vi "DataRootPathFGV.vi"(8 "Error In":errorcluster, 10 "action (write)":enum16{"write", "read"}(ring), 11 "PathIn":path) -> (0 "Error Out":errorcluster, 3 "PathOut":path)   [LabVIEW 2019]
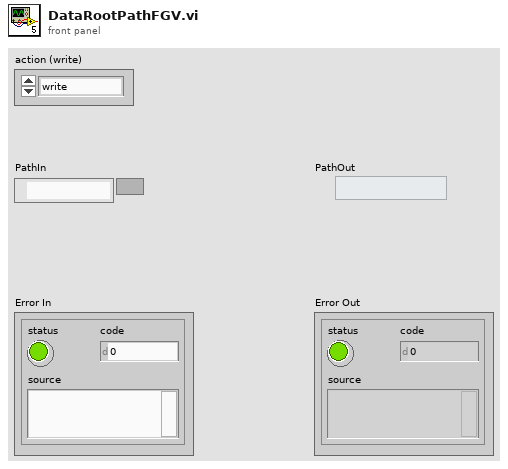
[diagram p1: front panel]
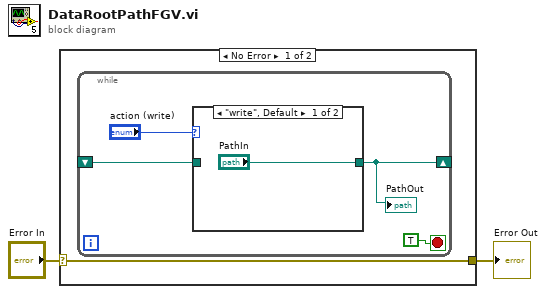
[diagram p0: block diagram]
diagram:
  n1 = case shown="No Error" "Error In" {
    selector: "Error In" -> [w3 w10]
    tunnel: [w3 w10] -> w1
    frame No Error {
      n2 = while {
        shift-right: [w6] -> _
        shift-left: _ -> [w4]
        stop <- TRUE stop-if-true
        n3 = case shown="\"write\", Default" "action (write)" {
          tunnel: ["PathIn" w9] -> w6
          tunnel: w4 -> [_ w9]
          frame "write", Default {
          }
          frame "read" {
          }
        }
        "PathOut" <- w6
      }
    }
    frame Error {
    }
  }
  "Error Out" <- w1
